vi "Application Control View.vi"(10 "User Events in":refnum<class "User Events.lvclass">) -> ()   [LabVIEW 2015, in "FAMT Views.lvlib"]
uses:
  FAMT Views.lvlib
  User Events/User Events.lvclass
  Commands/Command Factory/Command Factory.lvclass
  User Events/User Events.lvclass/User Events.ctl
  Typedefs/State Types.ctl
  Typedefs/Command Types.ctl
  Typedefs/FAMT Typedefs.lvlib
panel:
  in  "disableIsTrue":bool
  in  "enableIsTrue":bool
  in  "standbyIsTrue":bool
  in  "shutdownIsTrue":bool
  in  "startIsTrue":bool
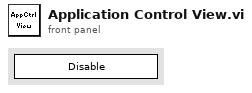
[diagram p1: front panel]
types:
  T1 = typedef "FAMT Typedefs.lvlib/Publish Data Events.ctl" = cluster{"State":refnum<user-event>, "ErrorCode":refnum<user-event>, "FC1 ILC Outputs":refnum<user-event>, "LogPath":refnum<user-event>, "FC1 ILC Inputs":refnum<user-event>, "Scan Progress":refnum<user-event>, "FC2 ILC Outputs":refnum<user-event>, "FC2 ILC Inputs":refnum<user-event>}
  T2 = typedef "FAMT Typedefs.lvlib/Subscribe Data Events.ctl" = cluster{"Command":refnum<user-event>}
  T3 = cluster{"Event Registration Refnum":refnum<event-registration>}
  T4 = typedef "FAMT Typedefs.lvlib/State Types.ctl" = enum16{"Offline State", "Fault State", "Standby State", "Disabled State", "Enabled State", "Wait For User Input State", "Perform Scan State"}
  T5 = typedef "FAMT Typedefs.lvlib/Command Types.ctl" = enum16{"Start", "Enable", "Disable", "Standby", "Shutdown", "Update"}
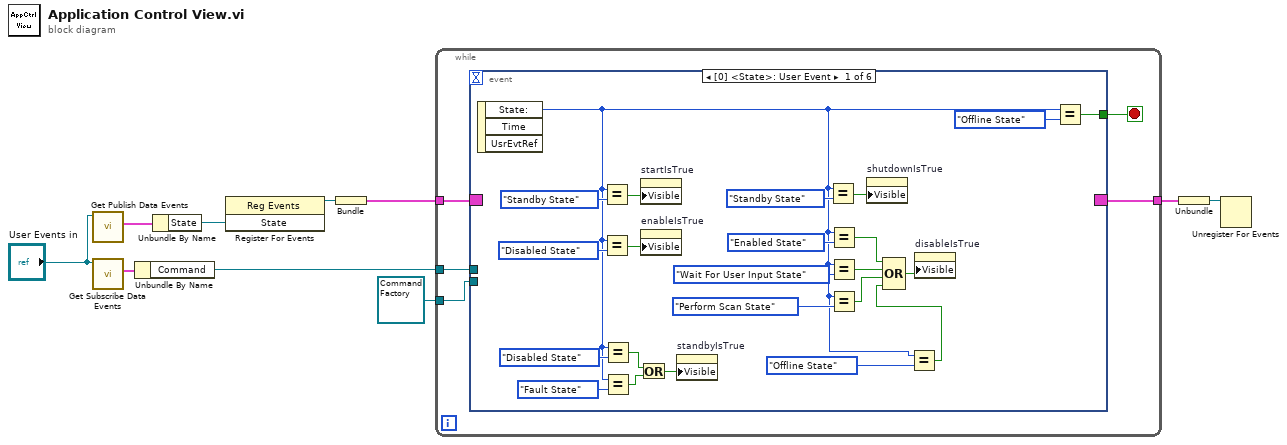
[diagram p0: block diagram]
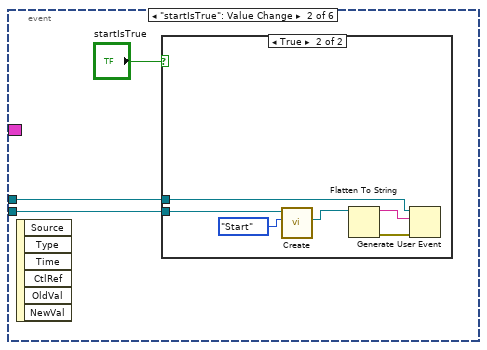
[diagram p2: hidden frame]
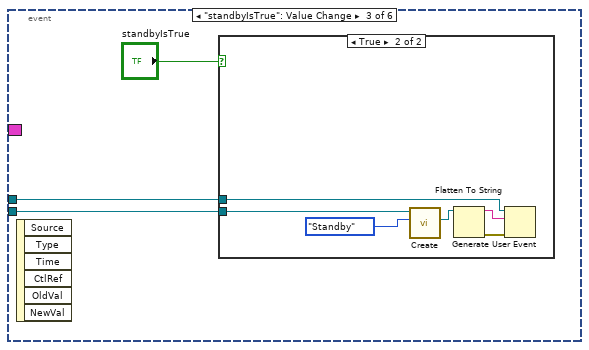
[diagram p4: hidden frame]
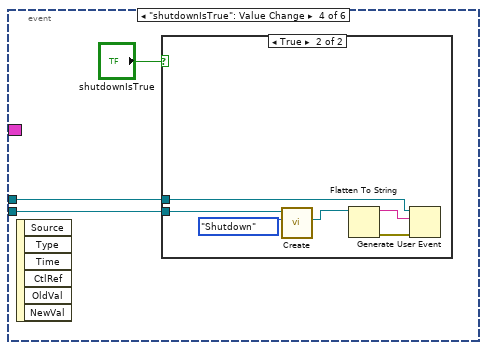
[diagram p6: hidden frame]
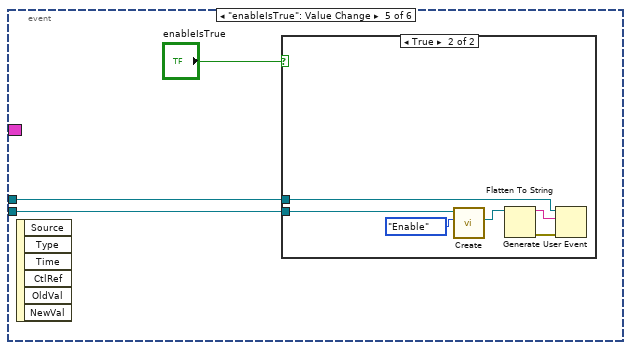
[diagram p8: hidden frame]
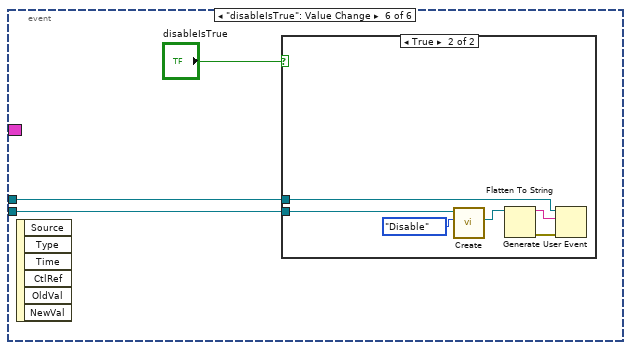
[diagram p10: hidden frame]
diagram:
  n1 = call "Get Publish Data Events.vi"("UserEvents in"="User Events in") -> ("Publish Data Events"=w7:T1)  [unwired: 9 in, 1 out]
  n2 = call "Get Subscribe Data Events.vi"("UserEvents in"="User Events in") -> ("Subscribe Data Events"=w8:T2)  [unwired: 9 in, 1 out]
  n3 = Unbundle By Name(w8) -> ("Command"=w5:refnum<user-event>)
  n4 = Unbundle By Name(w7) -> ("State"=w9:refnum<user-event>)
  n5 = register-events(w9) -> (reference out=w10:refnum<event-registration>)  [unwired: 2 in, 1 out]
  n6 = Bundle("Event Registration Refnum"=w10) -> (w6:T3)  [unwired: 1 in]
  n7 = while {
    tunnel: w6 -> [w15]
    tunnel: w5 -> [w14]
    tunnel: [w13] -> w4
    tunnel: refnum<class "Command Factory.lvclass"> refnum ("CommandFactory.lvclass") -> [w11]
    stop <- w12 stop-if-true
    n8 = event shown="[0] <State>: User Event" {
      selector: w15 -> [_ _ _ _ _ _]
      dyn-events: [_ _ _ _ _ _] -> w13
      timeout: _ -> [_ _ _ _ _ _]
      tunnel: w14 -> [_ w41 w49 w58 w67 w76]
      tunnel: [w37 _ _ _ _ _] -> w12
      tunnel: w11 -> [_ w40 w50 w59 w68 w77]
      event User Event {
        n9 = event-data() -> ("State:"=w17:T4)  [unwired: 1 in, 2 out]
        n10 = Equal?(x=w17, y=State_Types."Standby State") -> (x = y?=w35:bool)
        n11 = Equal?(x=w17, y=State_Types."Disabled State") -> (x = y?=w34:bool)
        n12 = Equal?(x=w17, y=State_Types."Disabled State") -> (x = y?=w29:bool)
        n13 = Equal?(x=w17, y=State_Types."Fault State") -> (x = y?=w30:bool)
        n14 = Or(x=w29, y=w30) -> (x .or. y?=w28:bool)
        n15 = property on="startIsTrue" class="Bool"("Visible"=w35) -> ()  [unwired: 2 in, 2 out]
        n16 = property on="enableIsTrue" class="Bool"("Visible"=w34) -> ()  [unwired: 2 in, 2 out]
        n17 = property on="standbyIsTrue" class="Bool"("Visible"=w28) -> ()  [unwired: 2 in, 2 out]
        n18 = Equal?(x=w17, y=State_Types."Standby State") -> (x = y?=w27:bool)
        n19 = Equal?(x=w17, y=State_Types."Enabled State") -> (x = y?=w20:bool)
        n20 = Equal?(x=w17, y=State_Types."Wait For User Input State") -> (x = y?=w21:bool)
        n21 = Equal?(x=w17, y=State_Types."Perform Scan State") -> (x = y?=w22:bool)
        n22 = property on="shutdownIsTrue" class="Bool"("Visible"=w27) -> ()  [unwired: 2 in, 2 out]
        n23 = Equal?(x=w17, y=State_Types."Offline State") -> (x = y?=w16:bool)
        n24 = Compound Arithmetic op=OR(w20, w21, w22, w16) -> (w19:bool)
        n25 = property on="disableIsTrue" class="Bool"("Visible"=w19) -> ()  [unwired: 2 in, 2 out]
        n26 = Equal?(x=w17, y=State_Types."Offline State") -> (x = y?=w37:bool)
      }
      event "startIsTrue": Value Change {
        n27 = event-data() -> ()  [unwired: 1 in, 6 out]
        n28 = case shown="True" "startIsTrue" {
          tunnel: w40 -> [_ w47]
          tunnel: w41 -> [_ w43]
          frame False {
          }
          frame True {
            n29 = call-dynamic "Create.vi"("Command Types"=Command_Types."Start" ("Command"), "Command Factory in"=w47) -> ("Command"=w42:refnum<class "Command.lvclass">)  [unwired: 7 in, 2 out]
            n30 = Flatten To String(anything=w42) -> (data string=w44:string, error out=w45:errorcluster)  [unwired: 3 in, 1 out]
            n31 = Generate User Event(user event=w43, event data cluster=w44, error in=w45) -> ()  [unwired: 1 in, 2 out]
          }
        }
      }
      event "standbyIsTrue": Value Change {
        n32 = event-data() -> ()  [unwired: 1 in, 6 out]
        n33 = case shown="True" "standbyIsTrue" {
          tunnel: w50 -> [_ w56]
          tunnel: w49 -> [_ w52]
          frame False {
          }
          frame True {
            n34 = call-dynamic "Create.vi"("Command Types"=Command_Types."Standby" ("Command"), "Command Factory in"=w56) -> ("Command"=w51:refnum<class "Command.lvclass">)  [unwired: 7 in, 2 out]
            n35 = Flatten To String(anything=w51) -> (data string=w53:string, error out=w54:errorcluster)  [unwired: 3 in, 1 out]
            n36 = Generate User Event(user event=w52, event data cluster=w53, error in=w54) -> ()  [unwired: 1 in, 2 out]
          }
        }
      }
      event "shutdownIsTrue": Value Change {
        n37 = event-data() -> ()  [unwired: 1 in, 6 out]
        n38 = case shown="True" "shutdownIsTrue" {
          tunnel: w59 -> [_ w65]
          tunnel: w58 -> [_ w61]
          frame False {
          }
          frame True {
            n39 = call-dynamic "Create.vi"("Command Types"=Command_Types."Shutdown" ("Command"), "Command Factory in"=w65) -> ("Command"=w60:refnum<class "Command.lvclass">)  [unwired: 7 in, 2 out]
            n40 = Flatten To String(anything=w60) -> (data string=w62:string, error out=w63:errorcluster)  [unwired: 3 in, 1 out]
            n41 = Generate User Event(user event=w61, event data cluster=w62, error in=w63) -> ()  [unwired: 1 in, 2 out]
          }
        }
      }
      event "enableIsTrue": Value Change {
        n42 = event-data() -> ()  [unwired: 1 in, 6 out]
        n43 = case shown="True" "enableIsTrue" {
          tunnel: w68 -> [_ w74]
          tunnel: w67 -> [_ w70]
          frame False {
          }
          frame True {
            n44 = call-dynamic "Create.vi"("Command Types"=Command_Types."Enable" ("Command"), "Command Factory in"=w74) -> ("Command"=w69:refnum<class "Command.lvclass">)  [unwired: 7 in, 2 out]
            n45 = Flatten To String(anything=w69) -> (data string=w71:string, error out=w72:errorcluster)  [unwired: 3 in, 1 out]
            n46 = Generate User Event(user event=w70, event data cluster=w71, error in=w72) -> ()  [unwired: 1 in, 2 out]
          }
        }
      }
      event "disableIsTrue": Value Change {
        n47 = event-data() -> ()  [unwired: 1 in, 6 out]
        n48 = case shown="True" "disableIsTrue" {
          tunnel: w77 -> [_ w83]
          tunnel: w76 -> [_ w79]
          frame False {
          }
          frame True {
            n49 = call-dynamic "Create.vi"("Command Types"=Command_Types."Disable" ("Command"), "Command Factory in"=w83) -> ("Command"=w78:refnum<class "Command.lvclass">)  [unwired: 7 in, 2 out]
            n50 = Flatten To String(anything=w78) -> (data string=w80:string, error out=w81:errorcluster)  [unwired: 3 in, 1 out]
            n51 = Generate User Event(user event=w79, event data cluster=w80, error in=w81) -> ()  [unwired: 1 in, 2 out]
          }
        }
      }
    }
  }
  n52 = Unbundle(w4) -> ("Event Registration Refnum"=w3:refnum<event-registration>)
  n53 = Unregister For Events(event registration refnum=w3) -> ()  [unwired: 1 in, 1 out]
